vi "Set Center Freq.vi"(8 "error in (no error)":errorcluster, 10 "Center Frequency":u32, 11 "RTL-SDR in":refnum<class "RTL-SDR.lvclass">) -> (0 "error out":errorcluster, 1 "function return":i32, 3 "RTL-SDR out":refnum<class "RTL-SDR.lvclass">)   [LabVIEW 2015, in "RTL-SDR.lvclass"]
uses:
  RTL-SDR.lvclass
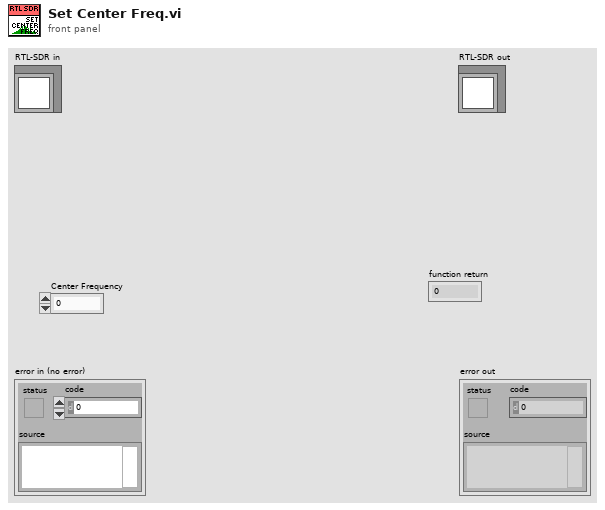
[diagram p1: front panel]
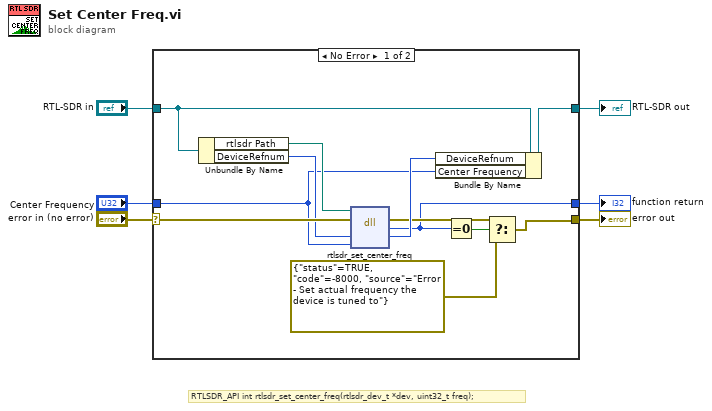
[diagram p0: block diagram]
diagram:
  # "RTLSDR_API int rtlsdr_set_center_freq(rtlsdr_dev_t *dev, uint32_t freq);"
  n1 = case shown="No Error" "error in (no error)" {
    selector: "error in (no error)" -> [w18 w20]
    tunnel: [w7 w20] -> w5
    tunnel: [w14 w19] -> w3
    tunnel: "RTL-SDR in" -> [w17 w19]
    tunnel: [w8 _] -> w2
    tunnel: "Center Frequency" -> [w12 _]
    frame No Error {
      n2 = Unbundle By Name(w17) -> ("rtlsdr Path"=w16:path, "DeviceRefnum"=w15:u64)
      n3 = dll-call lib="C:/Users/Ivan/Desktop/D-23-09-24 (RTL-SDR)/Project (Pelleng-SDR)/rtlsdr/dll/rtlsdr.*" fn="rtlsdr_set_center_freq"(path in=w16, error in=w18, "DeviceRefnum"=w15, "CenterFrequency"=w12) -> (error out=w9:errorcluster, "return type"=w8:i32, "DeviceRefnum"=w13:u64)  [unwired: 2 in, 1 out]
      n4 = Bundle By Name(cluster=w17, "DeviceRefnum"=w13, "Center Frequency"=w12) -> (w14:refnum<class "RTL-SDR.lvclass">)
      n5 = Equal To 0?(x=w8) -> (x = 0?=w10:bool)
      n6 = Select(t=w9, s=w10, f=errorcluster {"status"=TRUE, "code"=-8000, "source"="Error - Set actual frequency the device is tuned to"} ("error out")) -> (s? t:f=w7:errorcluster)
    }
    frame Error {
    }
  }
  "error out" <- w5
  "RTL-SDR out" <- w3
  "function return" <- w2
